vi "set Turntable Enabled.vi"(10 "Turntable Enabled":bool, 11 "Scene in":refnum<class "Scene.lvclass">) -> (3 "Scene out":refnum<class "Scene.lvclass">)   [LabVIEW 2020, in "Scene.lvclass"]
uses:
  Scene.lvclass
  Scene.lvclass/Scene.ctl
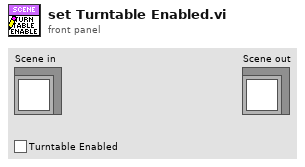
[diagram p1: front panel]
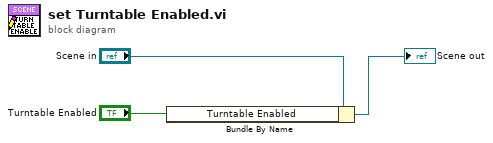
[diagram p0: block diagram]
diagram:
  n1 = Bundle By Name(cluster="Scene in", "Turntable Enabled"="Turntable Enabled") -> (→"Scene out":refnum<class "Scene.lvclass">)
